vi "Freefield-Config.vi"(0 "Cal Stimulus":T1, 7 "Speaker":string, 11 "error in (no error)":errorcluster, 12 "Path":path) -> (3 "Stimulus waveform":cluster{i32, dbl, dbl[]}, 4 "Stimulus":dbl[](array[numeric]), 8 "Mic Avg":dbl[][](array[numeric]), 10 "dt (ms)":dbl, 13 "df (Hz)":dbl, 15 "error out":errorcluster)   [LabVIEW 2020]
uses:
  In-Ear Calibration VIs/LV Source/Type Defs/Cal Stimulus.ctl
  epl-vi-lib/Connection VIs/Type Defs/CM-IO Type.ctl
  epl-vi-lib/PXI DAQ VIs/DAQ Engine VIs/AO Gain and Multiplier VIs/PXI Multipliers to AO Gains (1D).vi
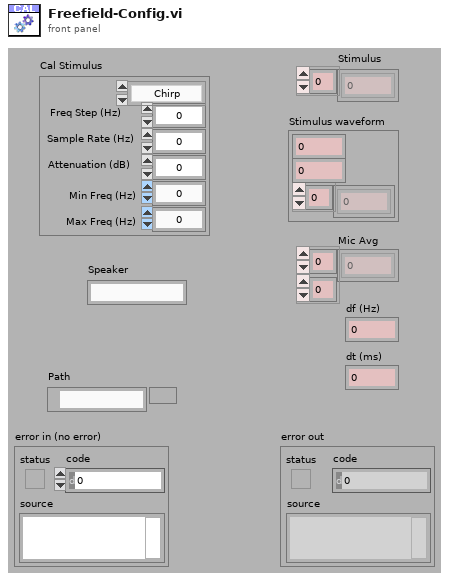
[diagram p1: front panel]
types:
  T1 = typedef "Cal Stimulus.ctl" = cluster{"Min Freq (Hz)":dbl, "Max Freq (Hz)":dbl, "Freq Step (Hz)":dbl, "Waveform":enum16{"Chirp", "Weighted"}, "Attenuation (dB)":dbl, "Sample Rate (Hz)":dbl}
  T2 = typedef "CM-IO Type.ctl" = enum16{"Analog Outputs", "Analog Inputs", "Digital Outputs", "Digital Inputs"}
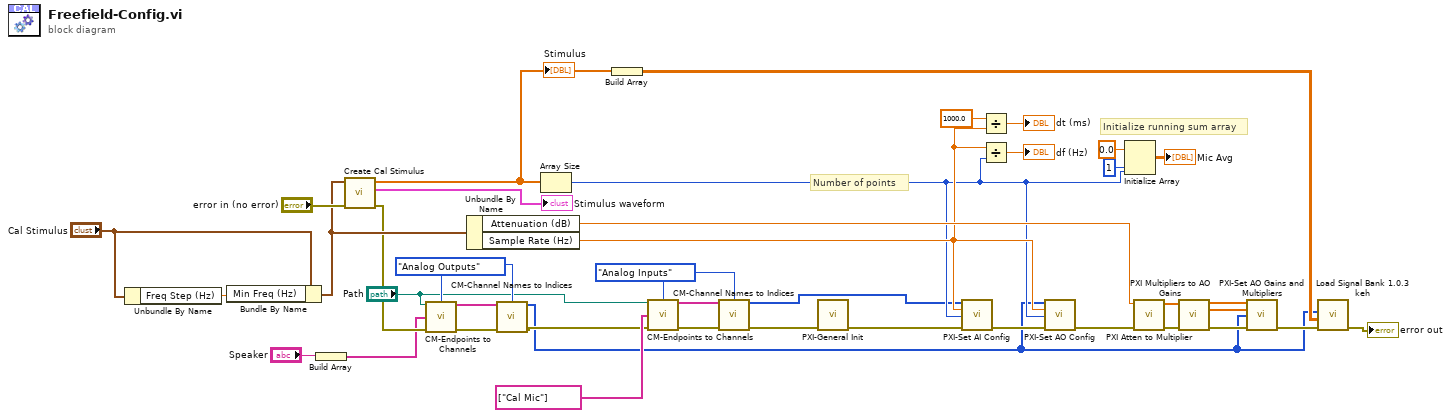
[diagram p0: block diagram]
diagram:
  w7 = CM-IO_Type."Analog Outputs" ("IO Type")
  w13 = CM-IO_Type."Analog Inputs" ("IO Type")
  # "Number of points"
  # "Initialize running sum array"
  n1 = Unbundle By Name("Cal Stimulus") -> ("Freq Step (Hz)"=w18:dbl)
  n2 = Bundle By Name(cluster="Cal Stimulus", "Min Freq (Hz)"=w18) -> (w16:T1)
  n3 = Build Array("Speaker") -> (w1:string[])
  n4 = call "Create Cal Stimulus.vi"("error in (no error)"="error in (no error)", "Cal Stimulus"=w16) -> ("error out"=w5:errorcluster, "Stimulus waveform"=→"Stimulus waveform":cluster{i32, dbl, dbl[]}, "Stimulus"=w40:dbl[])  [unwired: 7 in]
  "Stimulus" <- w40
  n5 = call "CM-Endpoints to Channels.vi"("Path"="Path", "IO Type"=w7, "Requested Endpoints"=w1, "error in (no error)"=w5) -> ("IO Channels"=w4:string[], "error out"=w9:errorcluster)  [unwired: 10 in]
  n6 = Unbundle By Name(w16) -> ("Attenuation (dB)"=w37:dbl, "Sample Rate (Hz)"=w21:dbl)
  n7 = call "CM-Channel Names to Indices.vi"("IO Channels"=w4, "IO Type"=w7, "error in (no error)"=w9) -> ("Indices"=w3:i32[], "error out"=w8:errorcluster)  [unwired: 11 in]
  n8 = Array Size(array=w40) -> (size(s)=w20:i32)
  n9 = Build Array(w40) -> (w19:dbl[][])
  n10 = call "CM-Endpoints to Channels.vi"("Path"="Path", "IO Type"=w13, "Requested Endpoints"=string[] ["Cal Mic"] ("Inputs"), "error in (no error)"=w8) -> ("IO Channels"=w14:string[], "error out"=w12:errorcluster)  [unwired: 10 in]
  n11 = call "CM-Channel Names to Indices.vi"("IO Channels"=w14, "IO Type"=w13, "error in (no error)"=w12) -> ("Indices"=w10:i32[], "error out"=w11:errorcluster)  [unwired: 11 in]
  n12 = call "PXI-General Init.vi"("error in (no error)"=w11) -> ("error out"=w26:errorcluster)  [unwired: 10 in]
  n13 = call "PXI-Set AI Config.vi"("AI Channels"=w10, "Sampling Rate (Hz)"=w21, "Buffer Size"=w20, "error in (no error)"=w26) -> ("error out"=w25:errorcluster)  [unwired: 11 in]
  n14 = Divide(x=1000.0, y=w21) -> (x/y=→"dt (ms)":dbl)
  n15 = Divide(x=w21, y=w20) -> (x/y=→"df (Hz)":dbl)
  n16 = call "PXI-Set AO Config.vi"("AO Channels"=w3, "Sampling Rate (Hz)"=w21, "Buffer Size"=w20, "error in (no error)"=w25) -> ("error out"=w24:errorcluster)  [unwired: 11 in]
  n17 = Initialize Array(0.0 ("element"), 1 ("dimension size"), w20) -> (→"Mic Avg":dbl[][])
  n18 = call "PXI Atten to Multiplier.vi"("error in (no error)"=w24, "Attenuation"=w37) -> ("error out"=w39:errorcluster, "Multiplier setting"=w38:dbl[])  [unwired: 8 in]
  n19 = call-poly "PXI Multipliers to AO Gains.vi"("Multipliers in"=w38, "error in (no error)"=w39) -> ("Multipliers out"=w23:dbl[], "Gains"=w22:dbl[], "error out"=w27:errorcluster)  [unwired: 11 in]
  n20 = call "PXI-Set AO Gains and Multipliers.vi"("Multipliers"=w23, "Gains"=w22, "AO Channels"=w3, "error in (no error)"=w27) -> ("error out"=w28:errorcluster)  [unwired: 11 in]
  n21 = call "Load Signal Bank 1.0.3 keh.vi"("error in (no error)"=w28, "Input array"=w19, "Active AO Array"=w3) -> ("error out"=→"error out":errorcluster)  [unwired: 6 in, 2 out]
